vi "toStringArray.vi"(8 "error in (no error)":errorcluster, 11 "RampUp in":refnum<class "RampUp.lvclass">) -> (0 "error out":errorcluster, 2 "eventStringArray":string[](array[string]), 3 "RampUp out":refnum<class "RampUp.lvclass">)   [LabVIEW 2011, in "Tools.lvlib" / "Scripting.lvlib" / "RampUp.lvclass"]
uses:
  RampUp.lvclass
  RampEvent/RampEvent.lvclass
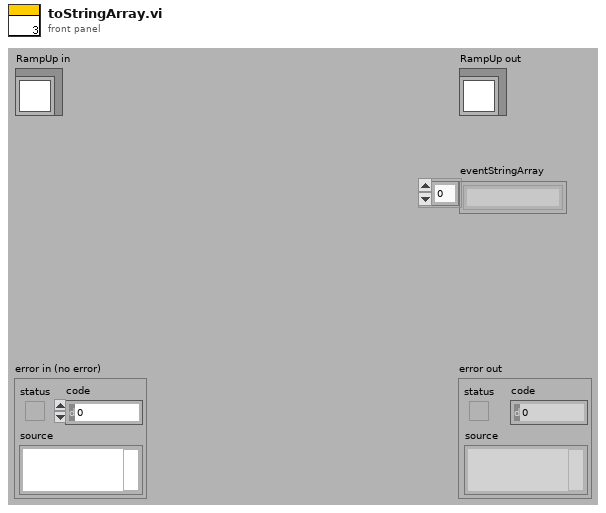
[diagram p1: front panel]
types:
  T1 = cluster{"rampTime":dbl, "timeStep":dbl, "dataValueStep":dbl}
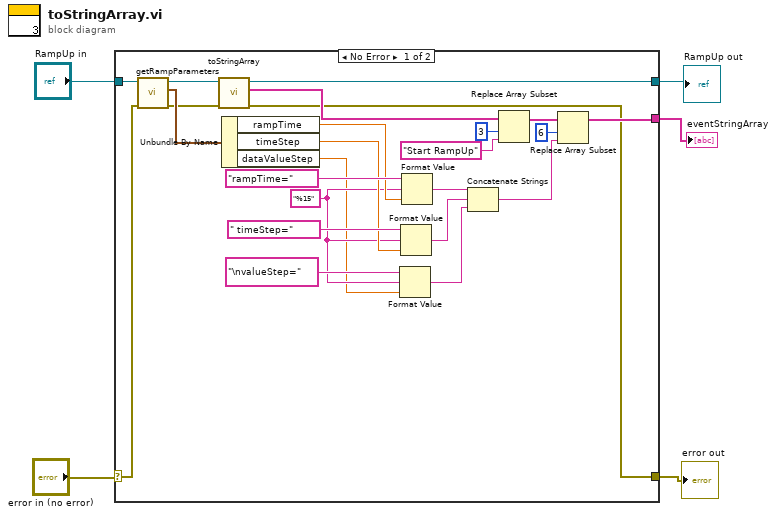
[diagram p0: block diagram]
diagram:
  n1 = case shown="No Error" "error in (no error)" {
    selector: "error in (no error)" -> [w7 w30]
    tunnel: "RampUp in" -> [w9 w31]
    tunnel: [w29 w31] -> w4
    tunnel: [w11 w30] -> w2
    tunnel: [w12 _] -> w1
    frame No Error {
      w23 = "%15"
      n2 = call "getRampParameters.vi"("error in (no error)"=w7, "RampEvent in"=w9) -> ("error out"=w6:errorcluster, "RampParameters"=w8:T1, "RampEvent out"=w10:refnum<class "RampUp.lvclass">)  [unwired: 7 in]
      n3 = call-parent "toStringArray.vi"("error in (no error)"=w6, "RampEvent in"=w10) -> ("error out"=w11:errorcluster, "eventStringArray"=w21:string[], "RampEvent out"=w29:refnum<class "RampUp.lvclass">)  [unwired: 7 in]
      n4 = Unbundle By Name(w8) -> ("rampTime"=w27:dbl, "timeStep"=w25:dbl, "dataValueStep"=w22:dbl)
      n5 = Format Value(string ("")="\nvalueStep=", format string=w23, value (0)=w22) -> (output string=w14:string)
      n6 = Format Value(string ("")=" timeStep=", format string=w23, value (0)=w25) -> (output string=w15:string)
      n7 = Format Value(string ("")="rampTime=", format string=w23, value (0)=w27) -> (output string=w16:string)
      n8 = Concatenate Strings(w16, w15, w14) -> (w13:string)
      n9 = Replace Array Subset(array=w21, new element="Start RampUp", index=3) -> (w19:string[])
      n10 = Replace Array Subset(array=w19, new element=w13, index=6) -> (w12:string[])
    }
    frame Error {
    }
  }
  "error out" <- w2
  "RampUp out" <- w4
  "eventStringArray" <- w1
